vi "Delete Goal.vi"(8 "error in (no error)":errorcluster, 10 "Category Summary":refnum<class "Expense Summary.lvclass">, 11 "Database in":refnum<class "Account History.lvclass">) -> (0 "error out":errorcluster, 3 "Database out":refnum<class "Account History.lvclass">)   [LabVIEW 2018, in "Account History.lvclass"]
uses:
  Account History.lvclass
  Expense Summary/Expense Summary.lvclass
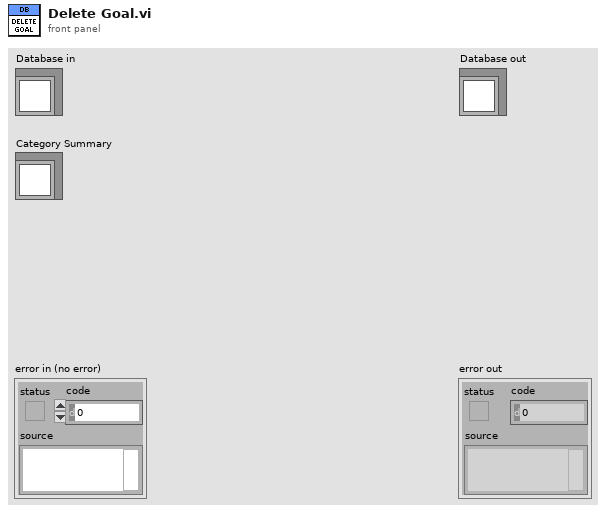
[diagram p1: front panel]
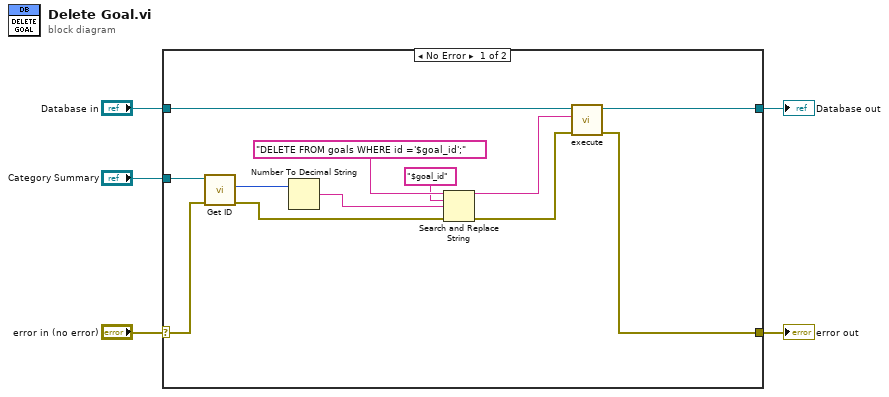
[diagram p0: block diagram]
diagram:
  n1 = case shown="No Error" "error in (no error)" {
    selector: "error in (no error)" -> [w7 w19]
    tunnel: [w12 w19] -> w4
    tunnel: [w16 w18] -> w2
    tunnel: "Database in" -> [w17 w18]
    tunnel: "Category Summary" -> [w9 _]
    frame No Error {
      n2 = call "Get ID.vi"("error in (no error)"=w7, "Expense Summary in"=w9) -> ("error out"=w6:errorcluster, "goal_id"=w8:i32)  [unwired: 7 in, 1 out]
      n3 = Number To Decimal String(number=w8) -> (decimal integer string=w10:string)  [unwired: 1 in]
      n4 = Search and Replace String(input string="DELETE FROM goals WHERE id ='$goal_id';", search string="$goal_id", replace string=w10, error in=w6) -> (result string=w14:string, error out=w13:errorcluster)  [unwired: 4 in, 2 out]
      n5 = call "execute.vi"("error in (no error)"=w13, "SQL query"=w14, "Database in"=w17) -> ("error out"=w12:errorcluster, "Database out"=w16:refnum<class "Account History.lvclass">)  [unwired: 7 in]
    }
    frame Error {
    }
  }
  "error out" <- w4
  "Database out" <- w2
